vi "TEST - Strip Units.vi"(8 "error in (no error)":errorcluster) -> (0 "error out":errorcluster, 2 "pass":bool)   [LabVIEW 2020, in "test_openg_variant.lvlib"]
uses:
  test_openg_variant.lvlib
  <userlib>/_OpenG.lib/error/error.llb/openg_error.lvlib
  source/library/openg_variant.lvlib
panel:
  out "Failures":T1(array[cluster])
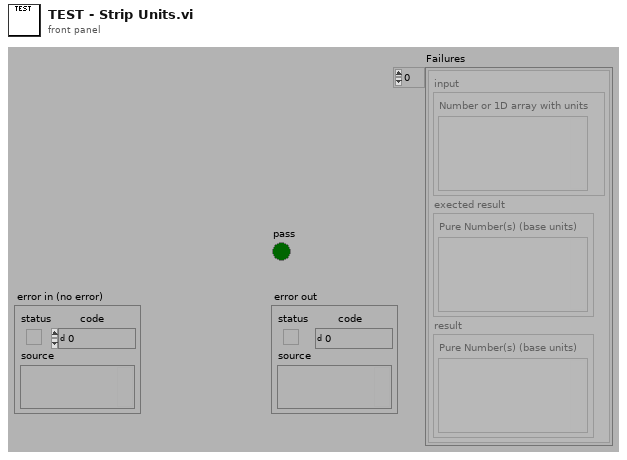
[diagram p1: front panel]
types:
  T1 = cluster{"input":cluster{"Number or 1D array with units":variant}, "exected result":cluster{"Pure Number(s) (base units)":variant}, "result":cluster{"Pure Number(s) (base units)":variant}}[]
  T2 = cluster{"input":cluster{"Number or 1D array with units":variant}, "exected result":cluster{"Pure Number(s) (base units)":variant}, "result":cluster{"Pure Number(s) (base units)":variant}}
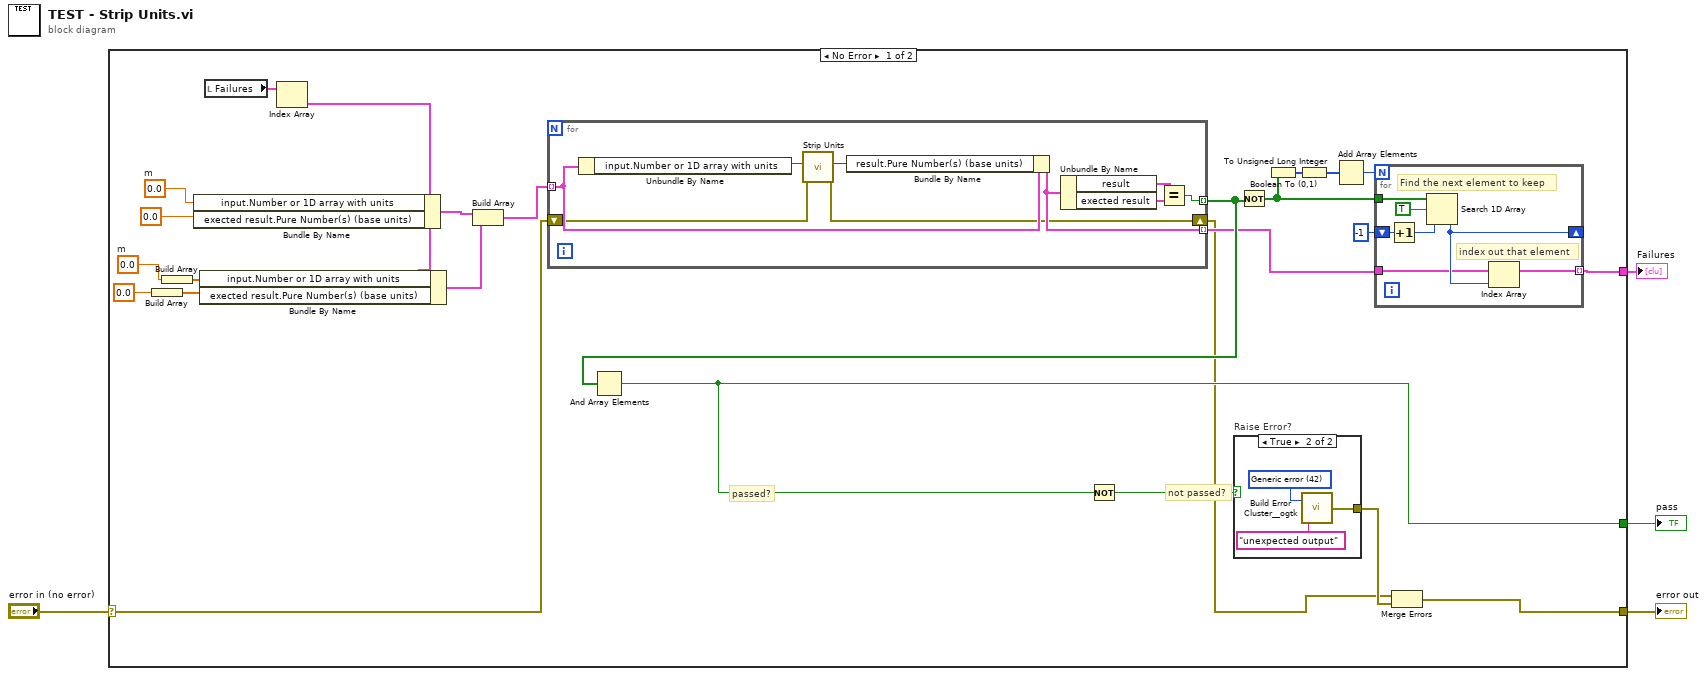
[diagram p0: block diagram]
diagram:
  n1 = case shown="No Error" "error in (no error)" {
    selector: "error in (no error)" -> [w15 w49]
    tunnel: [w26 _] -> w4
    tunnel: [w29 w49] -> w2
    tunnel: [w18 _] -> w1
    frame No Error {
      w8 = dbl[unit] 0.0  # m
      w11 = dbl[unit] 0.0  # m
      # "not passed?"
      # "passed?"
      n2 = Build Array(0.0) -> (w5:dbl[])
      n3 = Build Array(w8) -> (w6:dbl[unit][])
      n4 = local read "Failures"() -> (w13:T1)
      n5 = Index Array(array=w13) -> (element=w12:T2)  [unwired: 1 in]
      n6 = Bundle By Name(cluster=w12, "input.Number or 1D array with units"=w11, "exected result.Pure Number(s) (base units)"=0.0) -> (w17:T2)
      n7 = Bundle By Name(cluster=w12, "input.Number or 1D array with units"=w6, "exected result.Pure Number(s) (base units)"=w5) -> (w7:T2)
      n8 = Build Array(w17, w7) -> (w16:T1)
      n9 = for {
        tunnel: w16 -> [w44] mode=indexing
        tunnel: [w45] -> w20 mode=indexing
        tunnel: [w43] -> w19 mode=indexing
        shift-right: [w38] -> w14
        shift-left: w15 -> [w37]
        n10 = Unbundle By Name(w44) -> ("input.Number or 1D array with units"=w40:variant)
        n11 = call "Strip Units.vi"("error in (no error)"=w37, "Number or 1D array with units"=w40) -> ("error out"=w38:errorcluster, "Pure Number(s) (base units)"=w39:variant)  [unwired: 8 in]
        n12 = Bundle By Name(cluster=w44, "result.Pure Number(s) (base units)"=w39) -> (w43:T2)
        n13 = Unbundle By Name(w43) -> ("result"=w42:cluster{"Pure Number(s) (base units)":variant}, "exected result"=w41:cluster{"Pure Number(s) (base units)":variant})
        n14 = Equal?(x=w42, y=w41) -> (x = y?=w45:bool)
      }
      n15 = And Array Elements(Boolean array=w20) -> (logical AND=w26:bool)
      n16 = Not(x=w26) -> (.not. x?=w27:bool)
      n17 = case "Raise Error?" shown="True" w27 {
        tunnel: [_ w46] -> w28
        frame False {
        }
        frame True {
          w47 = 42 items=["No error", "Argument error", "Memory is full", "Out of zone", "End of file", "File already open", "Generic file I/O error", "File not found", "File permission error", "Disk is full", "Duplicate path", "Too many files open", "System feature not enabled", "Resource file not found", "Cannot add resource", "Resource not found", "Image not found", "Image memory error", "Pen does not exist", "Config type invalid", "Config token not found", "Config parse error", "Config memory error", "Bad external code format", "Bad external code offset", "External code not present", "Null window", "Destroy window error", "Null menu", "Print aborted", "Bad print record", "Print driver error", "Windows error during printing", "Memory error during printing", "Print dialog error", "Generic print error", "Invalid device refnum", "Device not found", "Device parameter error", "Device unit error", "Cannot open device", "Device call aborted", "Generic error", "Cancelled by user", "Object ID too low", "Object ID too high", "Object not in heap", "Unknown heap", "Unknown object (invalid DefProc)", "Unknown object (DefProc not in table)", "Message out of range", "Invalid (null) method", "Unknown message", "Manager call not supported", "Bad address", "Network operation in progress", "Network operation timed out", "Connection is busy", "Network attribute not supported", "Network error", "Address in use", "System out of memory", "Connection aborted", "Connection refused", "Not connected", "Already connected", "Connection closed", "Initialization error (interapplication manager)", "Bad occurrence", "Wait on unbound occurrence handler", "Occurrence queue overflow", "Datalog type conflict", "Unused", "Unrecognized type (interapplication manager)", "Memory corrupt", "Failed to make temporary DLL", "Old CIN version", "Drag socket not found", "Failed to load drop-object", "Failed to register OLE object", "Failed to release OLE object", "Format specifier type mismatch", "Unknown format specifier", "Too few format specifiers", "Too many format specifiers", "Scan failed", "Newer CIN version", "Error converting to variant", "Runtime menu error", "Password tampered", "Variant attribute not found", "Incompatible variant data type", "Event data is not available", "Event Store is not present", "Occurrence is not found", "Event Queue is not created", "Event info is not available", "Refnum passed is NULL", "Error retrieving Class GUID", "Error retrieving CoClass GUID", "Error retrieving TypeLib GUID.", "Bad built application magic bytes.", "Specific driver is different from the specific driver associated with the Logical Name.", "There is no session opened to the class driver.", "Max Error", "MAX - Error with config objects", "MAX - Error loading configuration", "MAX - Group not supported"]
          n18 = call <userlib>:"Build Error Cluster__ogtk.vi"("String to Prepend to source (\"\")"="unexpected output" ("String to Prepend to source (\"\")"), "code"=w47) -> ("error out"=w46:errorcluster)
        }
      }
      n19 = Not(x=w20) -> (.not. x?=w22:bool[])
      n20 = Boolean To (0,1)(Boolean=w22) -> (0, 1=w23:i16[])
      n21 = To Unsigned Long Integer(number=w23) -> (unsigned 32bit integer=w21:u32[])
      n22 = Add Array Elements(numeric array=w21) -> (sum=w24:u32)
      n23 = for {
        N: w24 -> [_]
        tunnel: w19 -> [w32]
        tunnel: w22 -> [w36]
        shift-right: [w33] -> _
        shift-left: -1 ("start index (0)") -> [w34]
        tunnel: [w31] -> w18 mode=indexing
        # "index out that element"
        # "Find the next element to keep"
        n24 = Increment(x=w34) -> (x+1=w30:i32)
        n25 = Search 1D Array(1D array=w36, element=TRUE, start index (0)=w30) -> (index of element=w33:i32)
        n26 = Index Array(array=w32, index=w33) -> (element=w31:T2)
      }
      n27 = Merge Errors(w14, w28) -> (w29:errorcluster)
    }
    frame Error {
    }
  }
  "pass" <- w4
  "error out" <- w2
  "Failures" <- w1
